vi "5數字加減.vi"() -> ()   [LabVIEW 2019]
panel:
  in  "Stop":bool
  out "N":i32
  in  "Dec":bool
  in  "Add":bool
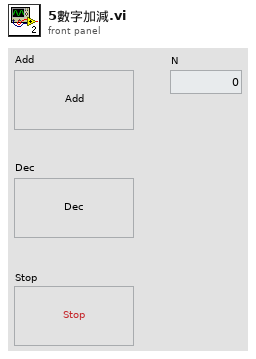
[diagram p1: front panel]
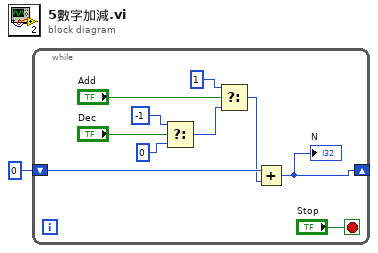
[diagram p0: block diagram]
diagram:
  n1 = while {
    shift-right: [w2] -> _
    shift-left: 0 ("N") -> [w4]
    stop <- "Stop" stop-if-true
    n2 = Select(t=-1 ("N"), s="Dec", f=0 ("N")) -> (s? t:f=w6:i32)
    n3 = Select(t=1 ("N"), s="Add", f=w6) -> (s? t:f=w3:i32)
    n4 = Add(x=w4, y=w3) -> (x+y=w2:i32)
    "N" <- w2
  }
